vi "qIDN.vi"(0 "System no.":i32=1 min=1 max=4 step=1, 5 "error in":errorcluster) -> (14 "Identification":string, 19 "error out":errorcluster)   [LabVIEW 2026]
doc: "GCS 3.0\n=====\n\n*IDN? (Get Device Identification)\n\nDescription \nQueries the device identification string.\n\nFormat\n*IDN?\n\nArguments\nnone\n\nResponse\nSingle-line text terminated by the line feed character, each component of which is separated by \na comma followed by a space. The text has the following format:\n<manufacturer>, <model>, <serial_number>, <firmware_rev_level>\n\nMeaning of the individual components:\n- <manufacturer> indicates the manufacturer and period of release. Default \"(c) <years> \nPhysik Instrumente (PI) SE & Co. KG\". May be shortened to \"(c) <years> PI\" in case \nof technical limitations. <years> follows (with a space) after (c) and must be specified as \na range in the form \"<year of first release> - <year of current release>\", e.g. \"(c) 2020 - \n2021\".\n- <model> indicates the exact product number of the device, e.g. \"E-880.2I1N\" and not \n\"E-880\".\n- <serial_number> indicates the serial number of the device.\n- <firmware_rev_level> indicates the version in the form <major version number>.<minor \nversion number>.<revision number>.<build number>, e.g. \"0.31.0.0\". Corresponds to \nthe APP information in the response to the VER? command. \n\nExample\n>>*IDN?\n<<(c) 2020 - 2021 Physik Instrumente (PI) SE & Co. KG, E880.2I1N, 120063890, 0.31.0.0\n\nNotes\nThe VER? command queries the versions of the firmware and other components such as drivers \nand libraries.\n\nUser command level\nUSR\n\n\nGCS 2.0\n=====\n\nReturns system identification string.\n\nE-816: This command cannot be issued to a slave."
panel:
  # "*IDN? (Get Device Identification)\n\nQueries the device identification string."
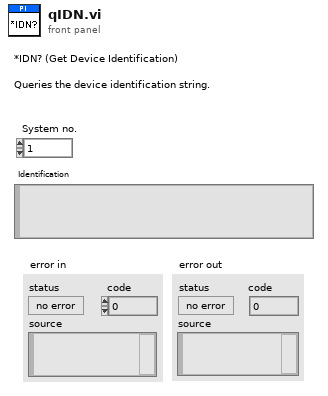
[diagram p1: front panel]
types:
  T1 = enum16{"Disable error check", "Force error check", "Use global settings"}
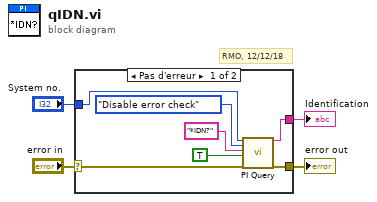
[diagram p0: block diagram]
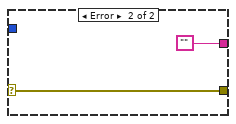
[diagram p2: hidden frame]
diagram:
  # "RMO, 12/12/18"
  n1 = case shown="Pas d'erreur" "error in" {
    selector: "error in" -> [w8 w13]
    tunnel: "System no." -> [w11 _]
    tunnel: [w10 ""] -> w3
    tunnel: [w9 w13] -> w2
    frame No Error {
      n2 = call "PI Query.vi"("System no."=w11, "Error check settings"=T1."Disable error check", "String to send"="*IDN?" ("String to Send"), "Attach termination char.?"=TRUE ("Attach Linefeed?"), "error in"=w8) -> ("String read"=w10:string, "error out"=w9:errorcluster)  [unwired: 2 in, 11 out]
    }
    frame Error {
    }
  }
  "Identification" <- w3
  "error out" <- w2
